vi "Get Windows User Name.vi"(8 "Error In":errorcluster) -> (0 "Error Out":errorcluster, 3 "User Name":string)   [LabVIEW 2021]
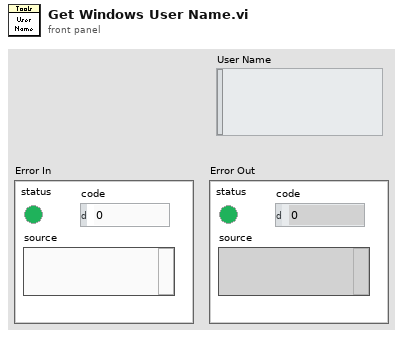
[diagram p1: front panel]
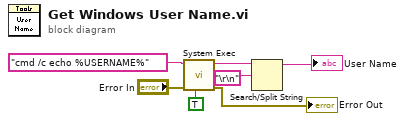
[diagram p0: block diagram]
diagram:
  n1 = call <vilib>:"System Exec.vi"("run minimized? (F)"=TRUE, "error in (no error)"="Error In", "command line"="cmd /c echo %USERNAME%") -> ("error out"=→"Error Out":errorcluster, "standard output"=w2:string)  [unwired: 5 in, 2 out]
  n2 = Search/Split String(string=w2, search string/char (-)="\r\n") -> (substring before match=→"User Name":string)  [unwired: 1 in, 2 out]
